vi "Finalize.vi"(8 "error in (no error)":errorcluster, 11 "Trigger in":refnum<class "Trigger.lvclass">) -> (0 "error out":errorcluster, 3 "Trigger out":refnum<class "Trigger.lvclass">)   [LabVIEW 2015, in "Trigger.lvclass"]
uses:
  Trigger.lvclass
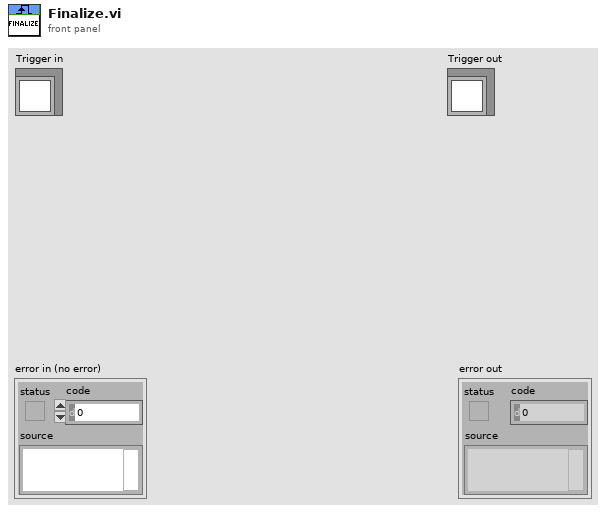
[diagram p1: front panel]
types:
  T1 = typedef "Trigger.lvclass/Trigger Type.ctl" = enum16{"Default", "Digital Edge", "Analog Edge", "In Range", "Value Change", "Boolean Evaluation"}
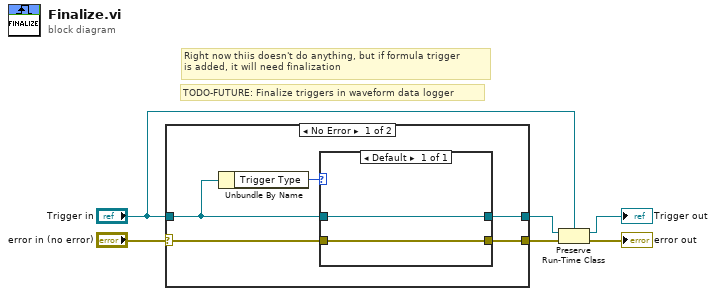
[diagram p0: block diagram]
diagram:
  # "TODO-FUTURE: Finalize triggers in waveform data logger"
  # "Right now thiis doesn't do anything, but if formula trigger\nis added, it will need finalization"
  n1 = case shown="No Error" "error in (no error)" {
    selector: "error in (no error)" -> [w8 w14]
    tunnel: "Trigger in" -> [w10 w15]
    tunnel: [w9 w15] -> w2
    tunnel: [w7 w14] -> w5
    frame No Error {
      n2 = Unbundle By Name(w10) -> ("Trigger Type"=w11:T1)
      n3 = case shown="Default" w11 {
        tunnel: w10 -> [w13]
        tunnel: [w13] -> w9
        tunnel: [w12] -> w7
        tunnel: w8 -> [w12]
        frame Default {
        }
      }
    }
    frame Error {
    }
  }
  n4 = Preserve Run-Time Class(object in=w2, error in=w5, 2:"Trigger in") -> (object out=→"Trigger out":refnum<class "Trigger.lvclass">, error out=→"error out":errorcluster)
